vi "Servo Pulse Gen._2.vi"() -> ()   [LabVIEW 2015]
uses:
  Galobal variable_TI.vi
  Project Setup/Globle Variable/GR_Servo.vi
  LCD Pressing Servo.ctl
panel:
  out "Servo _Motor2":T1
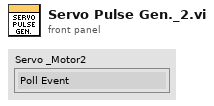
[diagram p1: front panel]
types:
  T1 = typedef "LCD Pressing Servo.ctl" = enum16{"Poll Event", "LCD  Press ServoCMD", "LCD Press Servo Home", "Exit"}
  T2 = cluster{"Emergency":bool, "Air Pressure":bool, "Saftey Sensor":bool, "Slide Servo  fault":bool, "LCD Pressing  Servo  fault":bool}
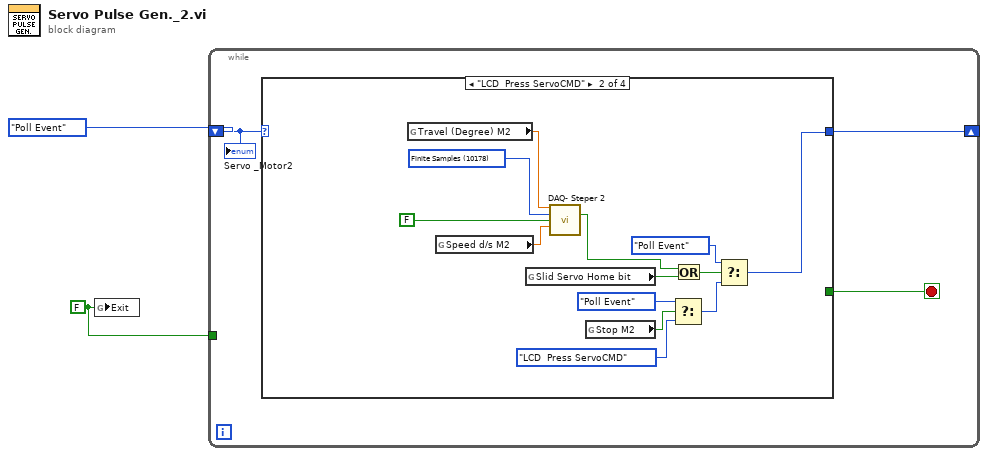
[diagram p0: block diagram]
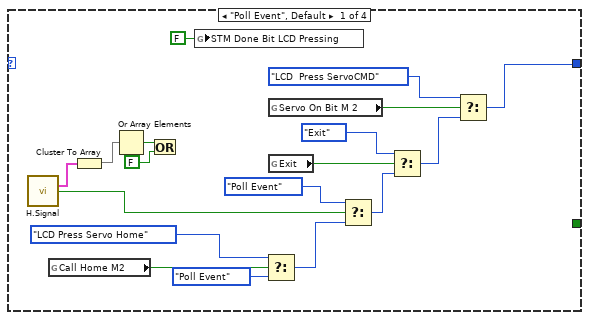
[diagram p2: hidden frame]
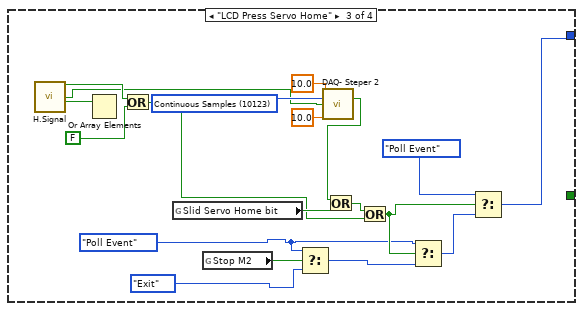
[diagram p3: hidden frame]
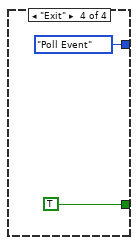
[diagram p4: hidden frame]
diagram:
  w1 = FALSE ("Exit")
  n1 = global write "Galobal variable_TI.vi" "Exit"(w1) -> ()
  n2 = while {
    shift-right: [w4] -> _
    shift-left: LCD_Pressing_Servo."Poll Event" ("Servo _Motor2") -> [w5]
    tunnel: w1 -> [_]
    stop <- w3 stop-if-true
    n3 = case shown="\"LCD  Press ServoCMD\"" w5 {
      tunnel: [w12 w26 w38 LCD_Pressing_Servo."Poll Event" ("f")] -> w4
      tunnel: [_ _ _ TRUE] -> w3
      frame "Poll Event", Default {
        n4 = call "H.Signal.vi"() -> ("H.Signal"=w10:T2, "LCD Pressing servo home RS"=w11:bool)  [unwired: 11 in, 3 out]
        n5 = global read "Galobal variable_TI.vi" "Call Home M2"() -> (w17:bool)
        n6 = Cluster To Array(cluster=w10) -> (array=w9:bool[])
        n7 = Or Array Elements(Boolean array=w9) -> (logical OR=w8:bool)
        n8 = Or(x=w8, y=FALSE) -> ()  [unwired: 1 out]
        n9 = global write "GR_Servo.vi" "STM Done Bit LCD Pressing"(FALSE ("STM Done Bit LCD Pressing")) -> ()
        n10 = Select(t=LCD_Pressing_Servo."LCD Press Servo Home" ("Servo _Motor2"), s=w17, f=LCD_Pressing_Servo."Poll Event") -> (s? t:f=w14:T1)
        n11 = global read "GR_Servo.vi" "Servo On Bit M 2"() -> (w22:bool)
        n12 = global read "Galobal variable_TI.vi" "Exit"() -> (w21:bool)
        n13 = Select(t=LCD_Pressing_Servo."Poll Event" ("Servo _Motor2"), s=w11, f=w14) -> (s? t:f=w13:T1)
        n14 = Select(t=LCD_Pressing_Servo."Exit" ("Servo _Motor2"), s=w21, f=w13) -> (s? t:f=w19:T1)
        n15 = Select(t=LCD_Pressing_Servo."LCD  Press ServoCMD" ("Servo _Motor2"), s=w22, f=w19) -> (s? t:f=w12:T1)
      }
      frame "LCD  Press ServoCMD" {
        w24 = 10178 items=["Finite Samples"=10178, "Continuous Samples"=10123, "Hardware Timed Single Point"=12522] ("Mode")
        n16 = global read "GR_Servo.vi" "Travel (Degree) M2"() -> (w35:dbl)
        n17 = global read "GR_Servo.vi" "Speed d/s M2"() -> (w36:dbl)
        n18 = global read "Galobal variable_TI.vi" "Slid Servo Home bit"() -> (w27:bool)
        n19 = call "DAQ- Steper 2.vi"("Travel (Degree)"=w35, "Mode"=w24, "Home Done"=FALSE, "Speed d/s"=w36) -> ("Task Done Bit"=w25:bool)  [unwired: 10 in, 1 out]
        n20 = global read "Galobal variable_TI.vi" "Stop M2"() -> (w29:bool)
        n21 = Select(t=LCD_Pressing_Servo."Poll Event" ("Servo _Motor2"), s=w29, f=LCD_Pressing_Servo."LCD  Press ServoCMD" ("Servo _Motor2")) -> (s? t:f=w30:T1)
        n22 = Or(x=w25, y=w27) -> (x .or. y?=w28:bool)
        n23 = Select(t=LCD_Pressing_Servo."Poll Event" ("Servo _Motor2"), s=w28, f=w30) -> (s? t:f=w26:T1)
      }
      frame "LCD Press Servo Home" {
        w41 = LCD_Pressing_Servo."Poll Event" ("Servo _Motor2")
        w55 = 10123 items=["Finite Samples"=10178, "Continuous Samples"=10123, "Hardware Timed Single Point"=12522] ("Mode")
        n24 = call "H.Signal.vi"() -> ("Slide servo home RS"=w51:bool, "LCD Pressing servo home RS"=w49:bool, "Bool_H Sig"=w50:bool)  [unwired: 11 in, 2 out]
        n25 = Or Array Elements(Boolean array=w50) -> ()  [unwired: 1 out]
        n26 = Or(x=w51, y=FALSE) -> (x .or. y?=w37:bool)
        n27 = global read "Galobal variable_TI.vi" "Slid Servo Home bit"() -> (w48:bool)
        n28 = global read "Galobal variable_TI.vi" "Stop M2"() -> (w46:bool)
        n29 = Select(t=w41, s=w46, f=LCD_Pressing_Servo."Exit" ("Servo _Motor2")) -> (s? t:f=w44:T1)
        n30 = call "DAQ- Steper 2.vi"("Travel (Degree)"=10.0, "Mode"=w55, "Home Done"=w49, "Speed d/s"=10.0) -> ("Task Done Bit"=w39:bool)  [unwired: 10 in, 1 out]
        n31 = Or(x=w39, y=w48) -> (x .or. y?=w47:bool)
        n32 = Or(x=w47, y=w37) -> (x .or. y?=w45:bool)
        n33 = Select(t=w41, s=w45, f=w44) -> (s? t:f=w43:T1)
        n34 = Select(t=LCD_Pressing_Servo."Poll Event" ("Servo _Motor2"), s=w45, f=w43) -> (s? t:f=w38:T1)
      }
      frame "Exit" {
      }
    }
    "Servo _Motor2" <- w5
  }
